vi "test Add Find Remove Alias.vi"(8 "error in (no error)":errorcluster, 11 "TestCase in":refnum<class "Switch Scripting Unit Tests.lvclass">) -> (0 "error out":errorcluster, 3 "TestCase out":refnum<class "Switch Scripting Unit Tests.lvclass">)   [LabVIEW 2017, in "Switch Scripting.lvlib" / "Switch Scripting Unit Tests.lvclass"]
uses:
  Switch Scripting Unit Tests.lvclass
  Routing Channel/Alias Mapping.ctl
  Switch Scripting Unit Tests.lvclass/Switch Scripting Unit Tests.ctl
  <vilib>/addons/_JKI Toolkits/VI Tester/TestCase.llb/TestCase.lvclass
  Switch Scripting.lvlib
  C:/Program Files (x86)/National Instruments/LabVIEW 2017/vi.lib/addons/_JKI Toolkits/VI Tester/TestCase.llb/TestCase.lvclass
panel:
  in  "Save?":bool
  out "Output Filename":string
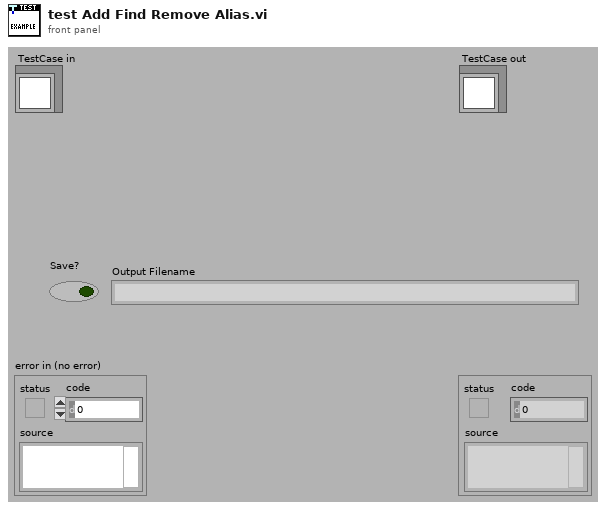
[diagram p1: front panel]
types:
  T1 = typedef "Switch Scripting.lvlib/Alias Mapping.ctl" = cluster{"alias":string, "pin":string}
  T2 = typedef "Custom Device API.lvlib/Custom Device Item Ref.ctl" = u64
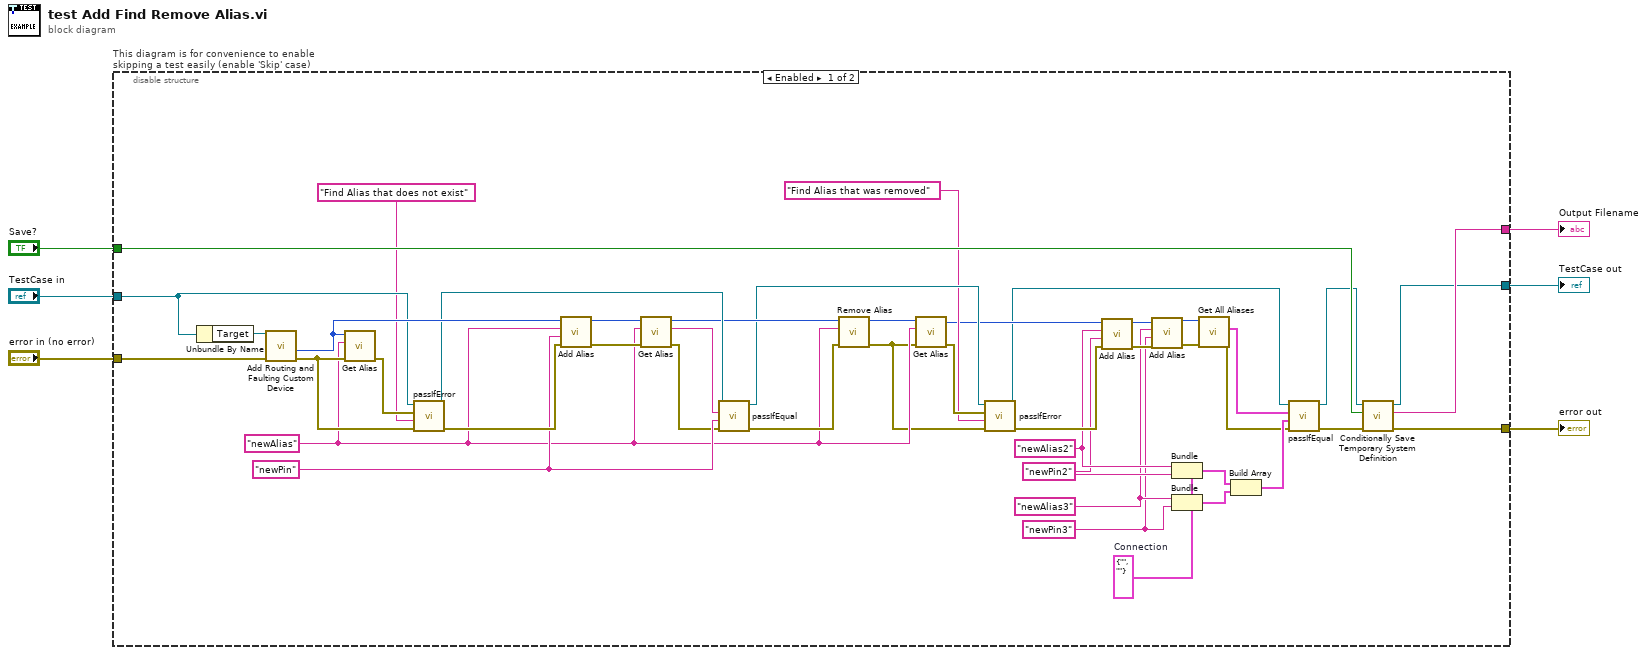
[diagram p0: block diagram]
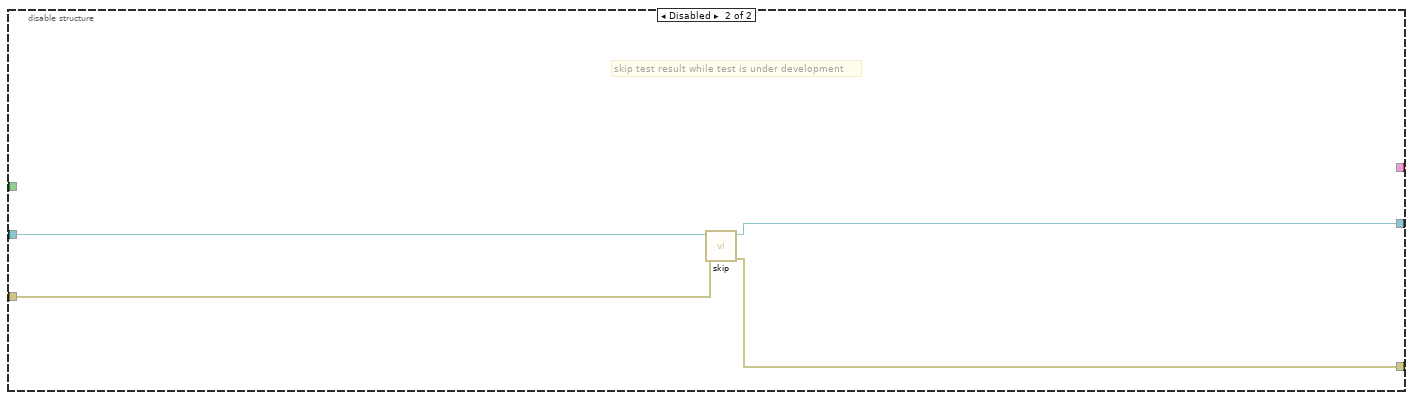
[diagram p2: hidden frame]
diagram:
  n1 = disable-structure "This diagram is for convenience to enable skipping a test easily (enable 'Skip' case)" shown="Enabled" {
    disable-tunnel: "TestCase in" -> [w44 w55]
    disable-tunnel: [w49 w53] -> w3
    disable-tunnel: [w50 w54] -> w5
    disable-tunnel: "error in (no error)" -> [w47 w52]
    disable-tunnel: [w51 _] -> w2
    disable-tunnel: "Save?" -> [w46 _]
    frame Enabled {
      w8 = T1 {"alias"="", "pin"=""}  # Connection
      w17 = "newPin3" ("Alias")
      w18 = "newAlias3" ("Alias")
      w19 = "newPin2" ("Alias")
      w20 = "newAlias2" ("Alias")
      w36 = "newPin" ("Pin")
      w27 = "newAlias" ("Alias")
      n2 = Unbundle By Name(w44) -> ("Target"=w48:refnum<k24>)
      n3 = call "Add Routing and Faulting Custom Device.vi"("error in (no error)"=w47, "Target in"=w48) -> ("error out"=w41:errorcluster, "Aliases Section Ref"=w45:T2)  [unwired: 5 in, 3 out]
      n4 = call "Get Alias.vi"("error in (no error)"=w41, "Alias"=w27, "Aliases Ref in"=w45) -> ("error out"=w43:errorcluster)  [unwired: 5 in, 3 out]
      n5 = call-dynamic "passIfError.vi"("error in (no error)"=w41, "task (\"\")"="Find Alias that does not exist" ("message (\"\")"), "error"=w43, "TestCase in"=w44) -> ("error out"=w40:errorcluster, "TestCase out"=w38:refnum<class "Switch Scripting Unit Tests.lvclass">)  [unwired: 6 in]
      n6 = call "Add Alias.vi"("error in (no error)"=w40, "Pin"=w36, "Alias"=w27, "Aliases Ref in"=w45) -> ("error out"=w34:errorcluster, "Aliases Ref out"=w39:T2)  [unwired: 6 in]
      n7 = call "Get Alias.vi"("error in (no error)"=w34, "Alias"=w27, "Aliases Ref in"=w39) -> ("error out"=w35:errorcluster, "Pin"=w37:string, "Aliases Ref out"=w33:T2)  [unwired: 5 in, 1 out]
      n8 = call-dynamic "passIfEqual.vi"("error in (no error)"=w35, "y"=w36, "x"=w37, "TestCase in"=w38) -> ("error out"=w29:errorcluster, "TestCase out"=w31:refnum<class "Switch Scripting Unit Tests.lvclass">)  [unwired: 6 in]
      n9 = call "Remove Alias.vi"("error in (no error)"=w29, "Alias"=w27, "Aliases Ref in"=w33) -> ("error out"=w7:errorcluster, "Aliases Ref out"=w30:T2)  [unwired: 6 in, 1 out]
      n10 = call "Get Alias.vi"("error in (no error)"=w7, "Alias"=w27, "Aliases Ref in"=w30) -> ("error out"=w32:errorcluster, "Aliases Ref out"=w26:T2)  [unwired: 5 in, 2 out]
      n11 = call-dynamic "passIfError.vi"("error in (no error)"=w7, "task (\"\")"="Find Alias that was removed" ("message (\"\")"), "error"=w32, "TestCase in"=w31) -> ("error out"=w25:errorcluster, "TestCase out"=w14:refnum<class "Switch Scripting Unit Tests.lvclass">)  [unwired: 6 in]
      n12 = call "Add Alias.vi"("error in (no error)"=w25, "Pin"=w19, "Alias"=w20, "Aliases Ref in"=w26) -> ("error out"=w24:errorcluster, "Aliases Ref out"=w23:T2)  [unwired: 6 in]
      n13 = call "Add Alias.vi"("error in (no error)"=w24, "Pin"=w17, "Alias"=w18, "Aliases Ref in"=w23) -> ("error out"=w21:errorcluster, "Aliases Ref out"=w22:T2)  [unwired: 6 in]
      n14 = Bundle(cluster=w8, "alias"=w20, "pin"=w19) -> (w16:T1)
      n15 = Bundle(cluster=w8, "alias"=w18, "pin"=w17) -> (w15:T1)
      n16 = call "Get All Aliases.vi"("error in (no error)"=w21, "Aliases Ref in"=w22) -> ("error out"=w10:errorcluster, "All Alias Mappings"=w12:T1[])  [unwired: 6 in, 2 out]
      n17 = Build Array(w16, w15) -> (w11:T1[])
      n18 = call-dynamic "passIfEqual.vi"("error in (no error)"=w10, "y"=w11, "x"=w12, "TestCase in"=w14) -> ("error out"=w9:errorcluster, "TestCase out"=w13:refnum<class "Switch Scripting Unit Tests.lvclass">)  [unwired: 6 in]
      n19 = call "Conditionally Save Temporary System Definition.vi"("error in (no error)"=w9, "Save?"=w46, "Test Case"=w13) -> ("error out"=w50:errorcluster, "filename"=w51:string, "Test Case"=w49:refnum<class "Switch Scripting Unit Tests.lvclass">)  [unwired: 6 in]
    }
    frame Disabled {
      # "skip test result while test is under development"
      n20 = call <vilib>:"skip.vi"("error in (no error)"=w52, "TestCase in"=w55) -> ("error out"=w54:errorcluster, "TestCase out"=w53:refnum<class "Switch Scripting Unit Tests.lvclass">)  [unwired: 8 in]
    }
  }
  "error out" <- w5
  "TestCase out" <- w3
  "Output Filename" <- w2
